vi "MakeItemVisible.vi"(0 "ListBox Ref In":refnum<vi>, 5 "Item Index":i32, 11 "Error In":errorcluster) -> (4 "ListBox Ref Out":refnum<vi>, 15 "Error Out":errorcluster)   [LabVIEW 2016, in "Drona.lvlib" / "ControlValue.lvlib" / "StimulusListbox.lvlib"]
doc: "Make the specified item index to visible in the listbox control."
uses:
  StimulusListbox.lvlib
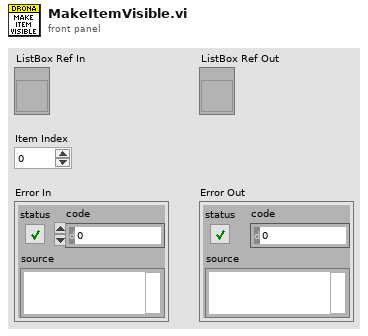
[diagram p1: front panel]
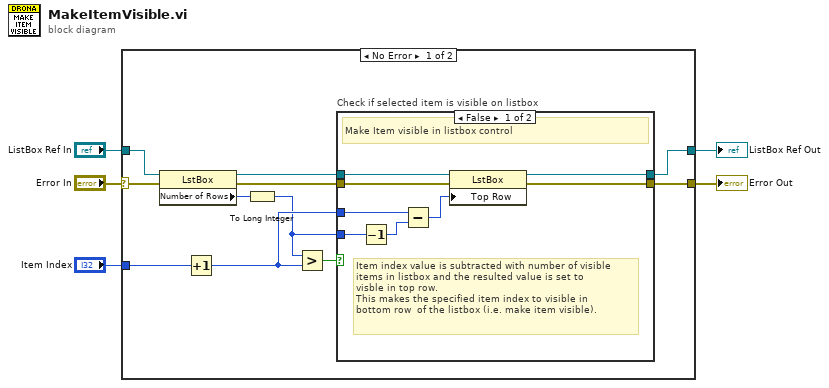
[diagram p0: block diagram]
diagram:
  n1 = case shown="No Error" "Error In" {
    selector: "Error In" -> [w6 w27]
    tunnel: [w16 w28] -> w5
    tunnel: "Item Index" -> [w15 _]
    tunnel: [w10 w27] -> w3
    tunnel: "ListBox Ref In" -> [w8 w28]
    frame No Error {
      n2 = property class="LstBox"(reference=w8, error in=w6) -> (reference out=w11:refnum<vi>, error out=w7:errorcluster, "Number of Rows"=w9:u32)
      n3 = Increment(x=w15) -> (x+1=w14:i32)
      n4 = To Long Integer(number=w9) -> (32bit integer=w12:i32)
      n5 = Greater?(x=w12, y=w14) -> (0:w13:bool)
      n6 = case "Check if selected item is visible on listbox" shown="False" w13 {
        tunnel: w7 -> [w24 w26]
        tunnel: [w23 w26] -> w10
        tunnel: w11 -> [w22 w25]
        tunnel: w14 -> [w21 _]
        tunnel: w12 -> [w20 _]
        tunnel: [w17 w25] -> w16
        frame False {
          # "Item index value is subtracted with number of visible \nitems in listbox and the resulted value is set to \nvisble in top row. \nThis makes the specified item index to visible in \nbottom row  of the listbox (i.e. make item visible)."
          # "Make Item visible in listbox control"
          n7 = Decrement(x=w20) -> (x-1=w18:i32)
          n8 = Subtract(x=w21, y=w18) -> (x-y=w19:i32)
          n9 = property class="LstBox"(reference=w22, error in=w24, "Top Row"=w19) -> (reference out=w17:refnum<vi>, error out=w23:errorcluster)
        }
        frame True {
          # "Specidied item index is already visible\non listbox"
        }
      }
    }
    frame Error {
    }
  }
  "ListBox Ref Out" <- w5
  "Error Out" <- w3
